vi "Get_values.vi"(4 "*Overflow":i16, 8 "error in (no error)":errorcluster, 10 "No Of Samples":i16, 11 "Handle":i16) -> (0 "error out":errorcluster, 1 "*Buffer_b":i16[](array[numeric]), 2 "*Buffer_a":i16[](array[numeric]), 3 "return type":i16)   [LabVIEW 2023]
uses:
  ps2000.dll
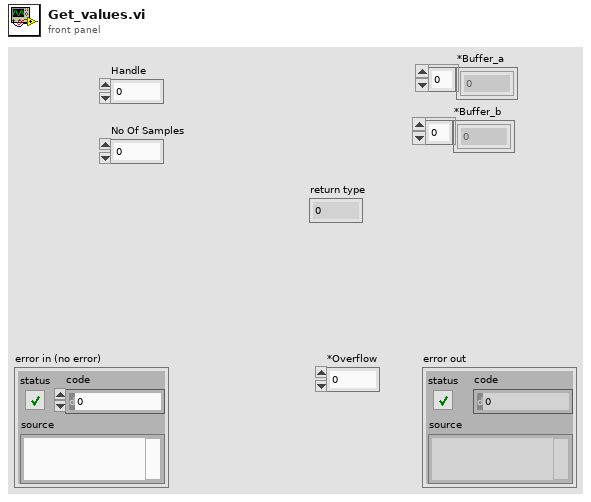
[diagram p1: front panel]
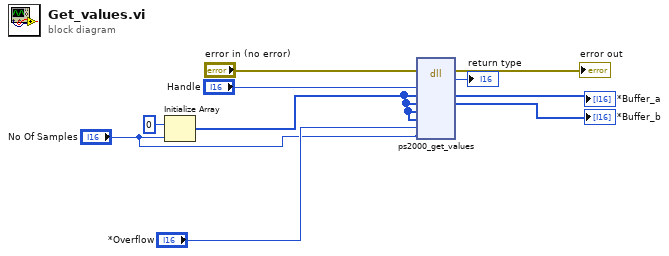
[diagram p0: block diagram]
diagram:
  n1 = Initialize Array(i8 0 ("element"), "No Of Samples") -> (w2:i8[])
  n2 = dll-call lib="C:/Users/cesar/Desktop/Ps2000 libreria/PS2000.dll" fn="ps2000_get_values"(error in="error in (no error)", "handle"="Handle", "*buffer_a"=w2, "*buffer_b"=w2, "*buffer_c"=w2, "*buffer_d"=w2, "*overflow"="*Overflow", "no_of_values"="No Of Samples") -> (error out=→"error out":errorcluster, "return type"=→"return type":i16, "*buffer_a"=→"*Buffer_a":i16[], "*buffer_b"=→"*Buffer_b":i16[])  [unwired: 7 in, 1 out]
